vi "Read Digitizer frequency.vi"(8 "error in (no error)":errorcluster, 11 "Combine_pulses in":refnum<class "Combine_pulses.lvclass">) -> (0 "error out":errorcluster, 2 "Digitizer frequency":dbl, 3 "Combine_pulses out":refnum<class "Combine_pulses.lvclass">)   [LabVIEW 2019, in "Combine_pulses.lvclass"]
uses:
  Combine_pulses.lvclass
  Combine_pulses.lvclass/Combine_pulses.ctl
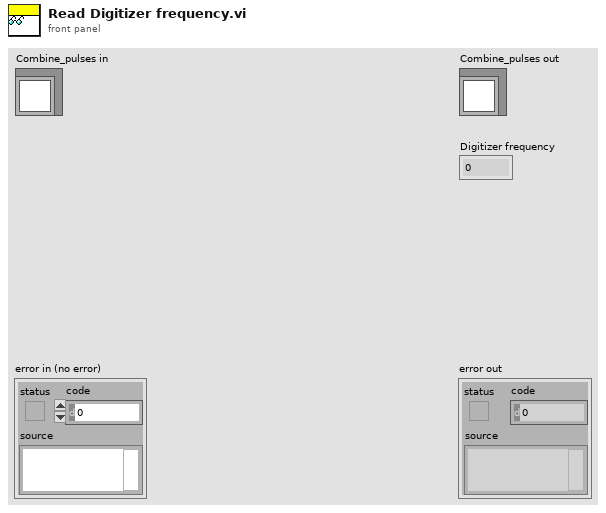
[diagram p1: front panel]
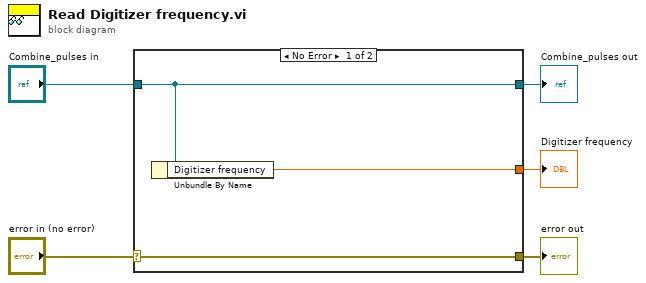
[diagram p0: block diagram]
diagram:
  n1 = case shown="No Error" "error in (no error)" {
    selector: "error in (no error)" -> [w8 w9]
    tunnel: [w8 w9] -> w4
    tunnel: [w7 w10] -> w2
    tunnel: "Combine_pulses in" -> [w7 w10]
    tunnel: [w6 _] -> w1
    frame No Error {
      n2 = Unbundle By Name(w7) -> ("Digitizer frequency"=w6:dbl)
    }
    frame Error {
    }
  }
  "error out" <- w4
  "Combine_pulses out" <- w2
  "Digitizer frequency" <- w1
